vi "Playback.vi"(8 "error in (no error)":errorcluster, 9 "vi path":path=path "E:/Scrubbing/sceneWindowPick.vi", 11 "Auto Folder Path":path=path "E:/Scrubbing/sceneWindowPick.vi") -> (0 "error out":errorcluster)   [LabVIEW 2013]
panel:
  out "Numeric 2":i32
  out "Array":path[](array[path])
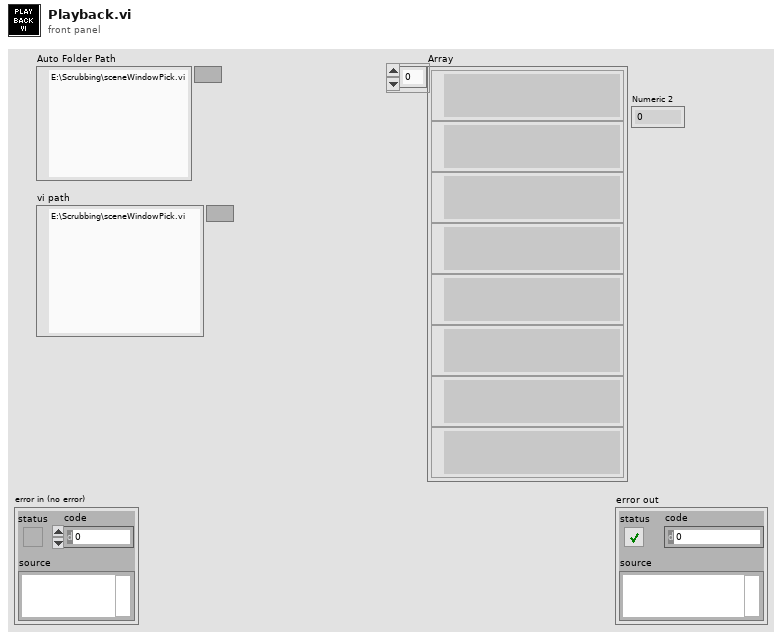
[diagram p1: front panel]
types:
  T1 = cluster{"Control labels for Images ?":string[], "Control Value:Get All":cluster{"Name":string, "Variant Data":variant}[]}
  T2 = typedef "imagedata.ctl" = cluster{"image type":i32, "image depth":i32, "image":u8[], "mask":u8[], "colors":u32[], "Rectangle":cluster{"left":i16, "top":i16, "right":i16, "bottom":i16}}
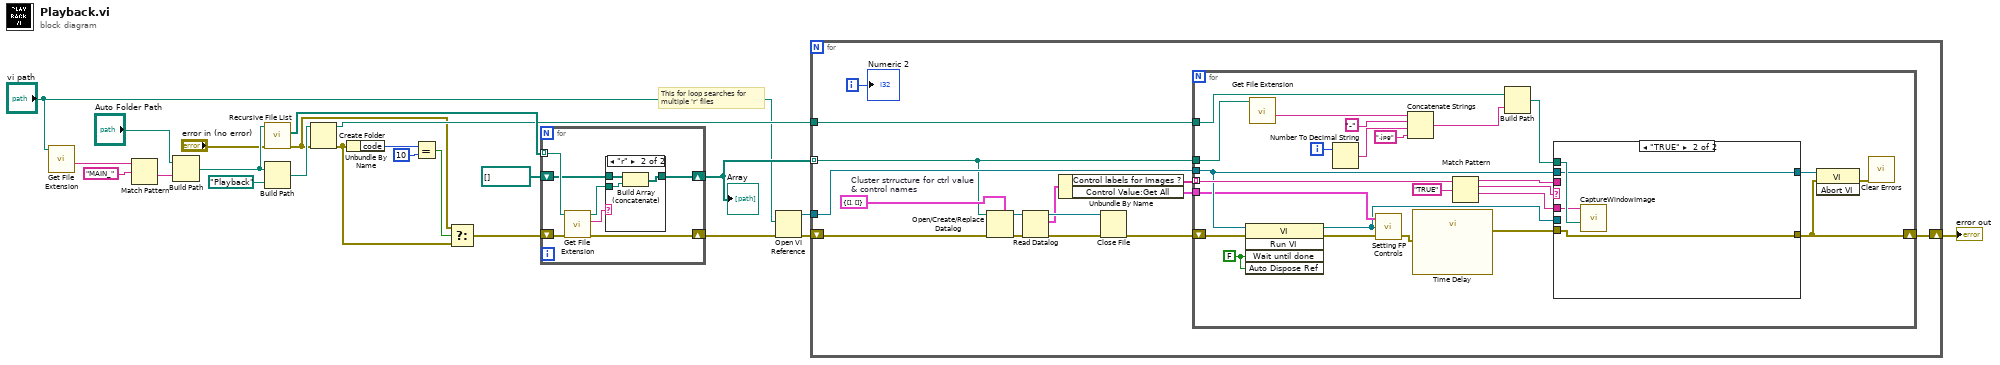
[diagram p0: block diagram]
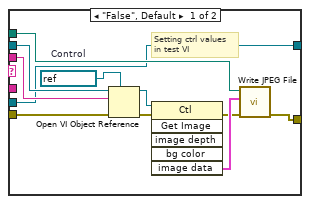
[diagram p2: hidden frame]
diagram:
  # "This for loop searches for \nmultiple 'r' files"
  n1 = call <vilib>:"Get File Extension.vi"("file"="vi path") -> ("filename without extension"=w10:string)  [unwired: 7 in, 3 out]
  n2 = Match Pattern(string=w10, regular expression="MAIN_") -> (after substring=w8:string)  [unwired: 1 in, 3 out]
  n3 = Build Path(base path="Auto Folder Path", name or relative path=w8) -> (appended path=w13:path)
  n4 = call <vilib>:"Recursive File List.vi"("error in (no error)"="error in (no error)", "Folder Path"=w13) -> ("error out"=w2:errorcluster, "All Files in Dir"=w23:path[])  [unwired: 5 in, 3 out]
  n5 = Build Path(base path=w13, name or relative path=path "Playback") -> (appended path=w17:path)
  n6 = Create Folder(path (use dialog)=w17, error in=w2) -> (created path=w16:path, error out=w3:errorcluster)  [unwired: 1 in, 1 out]
  n7 = Unbundle By Name(w3) -> ("code"=w6:i32)
  n8 = Equal?(x=w6, y=10) -> (x = y?=w4:bool)
  n9 = Select(t=w2, s=w4, f=w3) -> (s? t:f=w1:errorcluster)
  n10 = for {
    tunnel: w23 -> [w30] mode=indexing
    shift-right: [w27] -> w21
    shift-left: path[] [] -> [w26]
    shift-right: [w25] -> w7
    shift-left: w1 -> [w24]
    n11 = call <vilib>:"Get File Extension.vi"("error in (no error)"=w24, "file"=w30) -> ("error out"=w25:errorcluster, "lowercase file extension"=w29:string, "dup file"=w28:path)  [unwired: 6 in, 1 out]
    n12 = case shown="\"r\"" w29 {
      tunnel: w28 -> [_ w34]
      tunnel: [w31 w33] -> w27
      tunnel: w26 -> [w31 w32]
      frame "False", Default {
      }
      frame "r" {
        n13 = Build Array (concatenate)(w32, w34) -> (w33:path[])
      }
    }
  }
  "Array" <- w21
  n14 = Open VI Reference(vi path="vi path", error in (no error)=w7) -> (vi reference=w20:refnum<vi>, error out=w19:errorcluster)  [unwired: 4 in]
  n15 = for {
    tunnel: w21 -> [w39] mode=indexing
    tunnel: w20 -> [w44]
    shift-right: [w43] -> w11
    shift-left: w19 -> [w42]
    tunnel: w16 -> [w41]
    i -> [w45]
    w40 = T1 {"Control labels for Images ?"=[], "Control Value:Get All"=[]}  # Cluster strructure for ctrl value & control names
    n16 = Open/Create/Replace Datalog(5:w40, 8:w42, 11:w39) -> (0:w47:errorcluster, 3:w49:refnum<k1>)  [unwired: 3 in, 1 out]
    n17 = Read Datalog(4:w47, 7:w49) -> (0:w46:errorcluster, 2:w38:T1, 3:w48:refnum<k1>)  [unwired: 1 in]
    n18 = Unbundle By Name(w38) -> ("Control labels for Images ?"=w37:string[], "Control Value:Get All"=w35:cluster{"Name":string, "Variant Data":variant}[])
    n19 = Close File(refnum=w48, error in=w46) -> (error out=w36:errorcluster)  [unwired: 1 out]
    n20 = for {
      tunnel: w44 -> [w59]
      tunnel: w37 -> [w73] mode=indexing
      tunnel: w39 -> [w64]
      tunnel: w35 -> [w52]
      shift-right: [w55] -> w43
      shift-left: w36 -> [w57]
      tunnel: w41 -> [w63]
      i -> [w62]
      w58 = FALSE ("Wait Until Done")
      n21 = invoke class="VI" method="Run VI"(reference=w59, error in=w57, "Wait until done"=w58, "Auto Dispose Ref"=w58) -> (reference out=w51:refnum<vi>, error out=w54:errorcluster)  [unwired: 1 in, 3 out]
      n22 = call <vilib>:"Get File Extension.vi"("file"=w64) -> ("filename without extension"=w67:string)  [unwired: 7 in, 3 out]
      n23 = Number To Decimal String(number=w62) -> (decimal integer string=w66:string)  [unwired: 1 in]
      n24 = call "Setting FP Controls.vi"("error out"=w54, "This VI"=w51, "Control Value:Get All"=w52) -> ("error out 2"=w53:errorcluster)  [unwired: 2 in]
      n25 = Concatenate Strings(w67, "-" ("string"), w66, ".jpg" ("string")) -> (w68:string)
      n26 = call "Time Delay"("error in (no error)"=w53) -> ("error out"=w50:errorcluster)  [unwired: 10 in]
      n27 = Match Pattern(string=w73, regular expression="TRUE") -> (before substring=w60:string, match substring=w70:string, after substring=w72:string)  [unwired: 1 in, 1 out]
      n28 = Build Path(base path=w63, name or relative path=w68) -> (appended path=w61:path)
      n29 = case shown="\"TRUE\"" w70 {
        tunnel: w50 -> [w77 w86]
        tunnel: w59 -> [w82 w87]
        tunnel: w72 -> [_ w88]
        tunnel: [w78 w87] -> w71
        tunnel: [w75 w86] -> w55
        tunnel: w61 -> [w80 w89]
        tunnel: w60 -> [w79 _]
        tunnel: w51 -> [w78 _]
        frame "False", Default {
          w85 = refnum<vi> refnum  # Control
          # "Setting ctrl values\nin test VI"
          n30 = Open VI Object Reference(7:w85, 8:w77, 10:w79, 11:w82) -> (0:w81:errorcluster, 3:w84:refnum<vi>)
          n31 = invoke class="Ctl" method="Get Image"(reference=w84, error in=w81) -> (error out=w76:errorcluster, "image data"=w83:T2)  [unwired: 4 in, 4 out]
          n32 = call <vilib>:"Write JPEG File.vi"("error in (no error)"=w76, "image data"=w83, "path to JPEG file"=w80) -> ("error out"=w75:errorcluster)  [unwired: 7 in, 1 out]
        }
        frame "TRUE" {
          n33 = call "CaptureWindowImage.vi"("File Path"=w89, "Window Name"=w88) -> ()  [unwired: 9 in, 1 out]
        }
      }
      n34 = invoke class="VI" method="Abort VI"(reference=w71, error in=w55) -> (error out=w56:errorcluster)  [unwired: 1 in, 2 out]
      n35 = call <vilib>:"Clear Errors.vi"("error in (no error)"=w56) -> ()  [unwired: 6 in, 1 out]
    }
    "Numeric 2" <- w45
  }
  "error out" <- w11
